vi "csv_control_04.vi"(8 "error in (no error)":errorcluster caption="错误输入（无错误）", 9 "Low_Litmit":string, 10 "High_Litmit":string, 11 "SN":string) -> (0 "error out":errorcluster caption="错误输出", 2 "布尔":bool, 3 "output":string)   [LabVIEW 2024]
panel:
  in  "SN 2":string
  in  "Test_ID 2":string
  in  "Test_Value 2":dbl
  in  "Test_Value":dbl
  in  "Test_ID":string
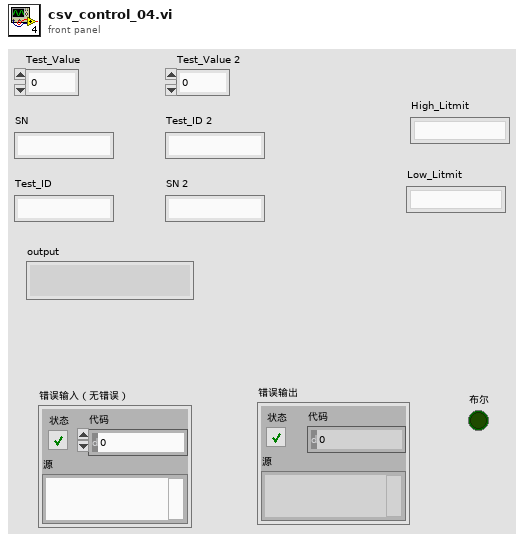
[diagram p1: front panel]
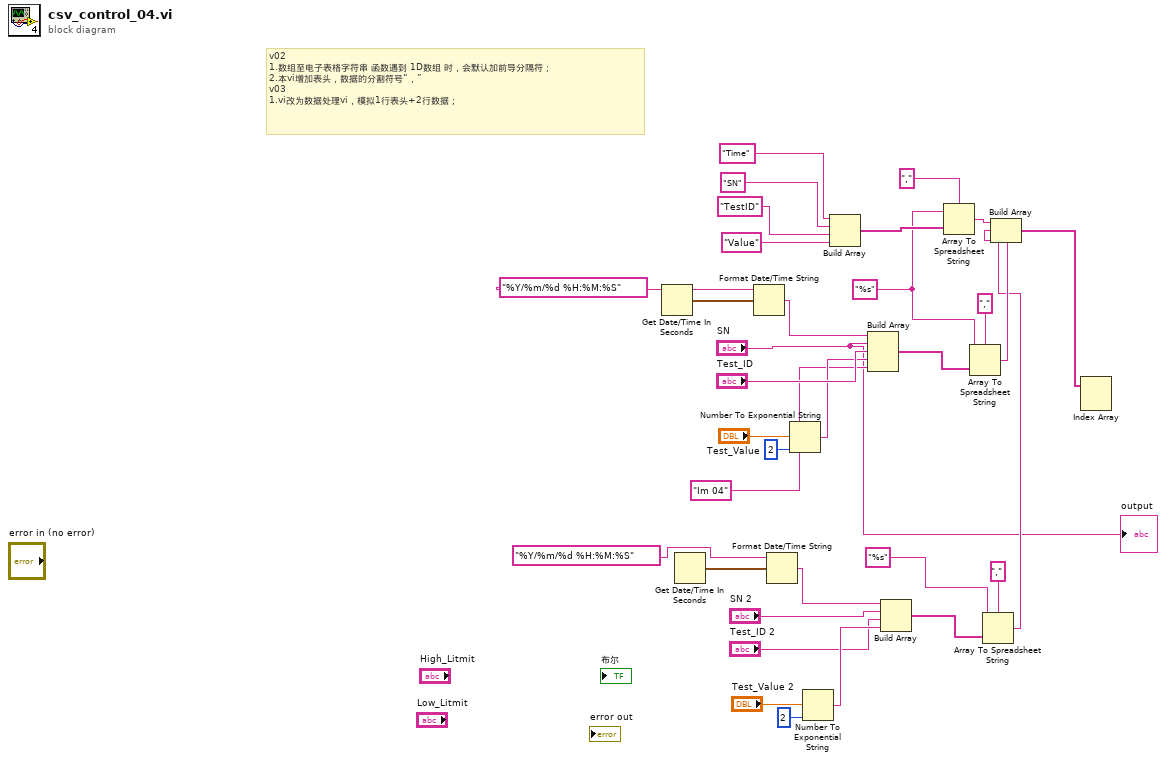
[diagram p0: block diagram]
diagram:
  w19 = "%s" ("格式字符串")
  # "v02\n1.数组至电子表格字符串 函数遇到 1D数组 时，会默认加前导分隔符；\n2.本vi增加表头，数据的分割符号“，”\nv03\n1.vi改为数据处理vi，模拟1行表头+2行数据；"
  n1 = Get Date/Time In Seconds() -> (seconds since 1Jan1904=w30:timestamp)
  n2 = Get Date/Time In Seconds() -> (seconds since 1Jan1904=w10:timestamp)
  n3 = Format Date/Time String(time format string (%c)="%Y/%m/%d %H:%M:%S" ("时间格式字符串(%c)"), seconds (now)=w30) -> (date/time string=w26:string)  [unwired: 1 in]
  n4 = Format Date/Time String(time format string (%c)="%Y/%m/%d %H:%M:%S" ("时间格式字符串(%c)"), seconds (now)=w10) -> (date/time string=w13:string)  [unwired: 1 in]
  n5 = Number To Exponential String(number="Test_Value", precision (6)=i16 2 ("精度(6)")) -> (E-format string=w31:string)  [unwired: 2 in]
  n6 = Number To Exponential String(number="Test_Value 2", precision (6)=i16 2 ("精度(6)")) -> (E-format string=w9:string)  [unwired: 2 in]
  n7 = Build Array("Time" ("元素"), "SN" ("元素"), "TestID" ("元素"), "Value" ("元素")) -> (w20:string[])
  n8 = Build Array(w26, "SN", "Test_ID", w31, "Im 04" ("元素")) -> (w28:string[])
  n9 = Build Array(w13, "SN 2", "Test_ID 2", w9) -> (w11:string[])
  n10 = Array To Spreadsheet String(delimiter (Tab)="," ("分隔符(Tab)"), array=w20, 3:w19) -> (spreadsheet string=w17:string)
  n11 = Array To Spreadsheet String(delimiter (Tab)="," ("分隔符(Tab)"), array=w28, 3:w19) -> (spreadsheet string=w16:string)
  n12 = Array To Spreadsheet String(delimiter (Tab)="," ("分隔符(Tab)"), array=w11, 3:"%s" ("格式字符串")) -> (spreadsheet string=w4:string)
  n13 = Build Array(w17, w16, w4) -> (w3:string[])
  n14 = Index Array(array=w3) -> ()  [unwired: 2 in, 2 out]
  "output" <- "SN"
